vi "extract ROI data.vi"(8 "error in (no error)":errorcluster, 11 "LineCCD in":refnum<class "LineCCD.lvclass">) -> (0 "error out":errorcluster, 3 "LineCCD out":refnum<class "LineCCD.lvclass">)   [LabVIEW 2012, in "LineCCD.lvclass"]
uses:
  LineCCD.lvclass
  LineCCD.lvclass/LineCCD.ctl
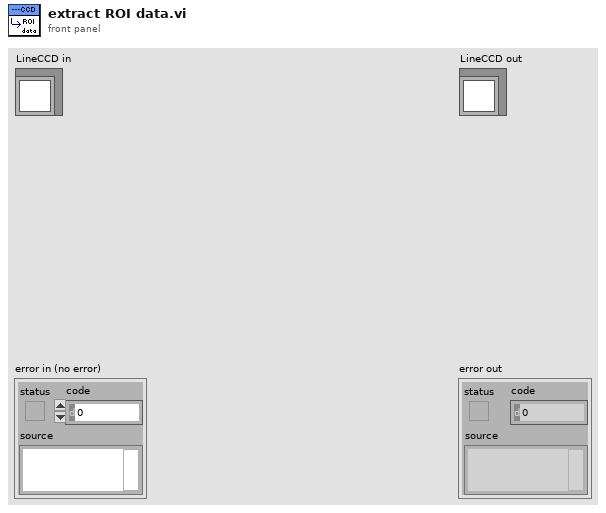
[diagram p1: front panel]
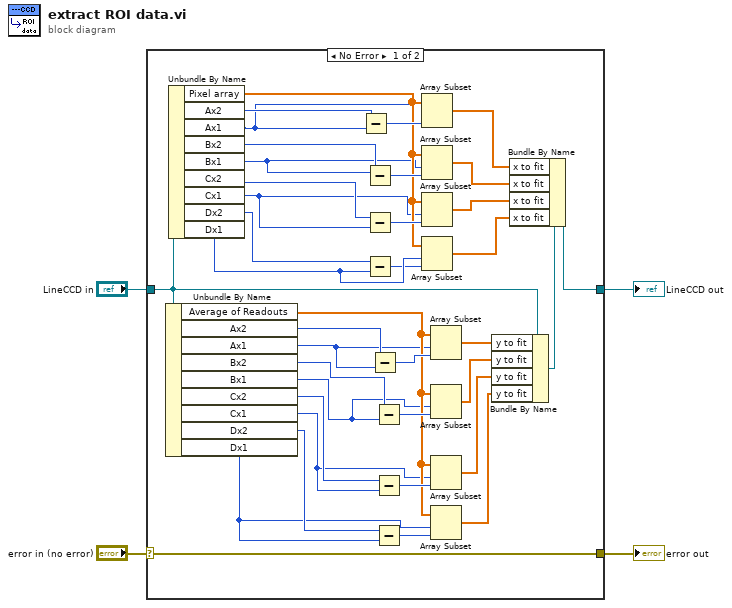
[diagram p0: block diagram]
diagram:
  n1 = case shown="No Error" "error in (no error)" {
    selector: "error in (no error)" -> [w42 w44]
    tunnel: [w42 w44] -> w3
    tunnel: [w9 w43] -> w1
    tunnel: "LineCCD in" -> [w24 w43]
    frame No Error {
      n2 = Unbundle By Name(w24) -> ("Average of Readouts"=w33:dbl[], "Ax2"=w32:i32, "Ax1"=w31:i32, "Bx2"=w30:i32, "Bx1"=w29:i32, "Cx2"=w28:i32, "Cx1"=w27:i32, "Dx2"=w26:i32, "Dx1"=w25:i32)
      n3 = Unbundle By Name(w24) -> ("Pixel array"=w20:dbl[], "Ax2"=w19:i32, "Ax1"=w18:i32, "Bx2"=w17:i32, "Bx1"=w16:i32, "Cx2"=w15:i32, "Cx1"=w14:i32, "Dx2"=w13:i32, "Dx1"=w12:i32)
      n4 = Subtract(x=w19, y=w18) -> (x-y=w21:i32)
      n5 = Subtract(x=w17, y=w16) -> (x-y=w22:i32)
      n6 = Subtract(x=w15, y=w14) -> (x-y=w23:i32)
      n7 = Subtract(x=w13, y=w12) -> (x-y=w11:i32)
      n8 = Subtract(x=w32, y=w31) -> (x-y=w41:i32)
      n9 = Subtract(x=w30, y=w29) -> (x-y=w40:i32)
      n10 = Subtract(x=w28, y=w27) -> (x-y=w39:i32)
      n11 = Subtract(x=w26, y=w25) -> (x-y=w38:i32)
      n12 = Array Subset(array=w20, index=w18, length=w21) -> (w8:dbl[])
      n13 = Array Subset(array=w20, index=w16, length=w22) -> (w7:dbl[])
      n14 = Array Subset(array=w20, index=w14, length=w23) -> (w6:dbl[])
      n15 = Array Subset(array=w20, index=w12, length=w11) -> (w5:dbl[])
      n16 = Array Subset(array=w33, index=w31, length=w41) -> (w37:dbl[])
      n17 = Array Subset(array=w33, index=w29, length=w40) -> (w36:dbl[])
      n18 = Array Subset(array=w33, index=w27, length=w39) -> (w35:dbl[])
      n19 = Array Subset(array=w33, index=w25, length=w38) -> (w34:dbl[])
      n20 = Bundle By Name(cluster=w24, "y to fit"=w37, "y to fit"=w36, "y to fit"=w35, "y to fit"=w34) -> (w10:refnum<class "LineCCD.lvclass">)
      n21 = Bundle By Name(cluster=w10, "x to fit"=w8, "x to fit"=w7, "x to fit"=w6, "x to fit"=w5) -> (w9:refnum<class "LineCCD.lvclass">)
    }
    frame Error {
    }
  }
  "error out" <- w3
  "LineCCD out" <- w1
